vi "Write Direction.vi"(10 "Velocity":T1, 11 "Flying Saucer in":refnum<class "Flying Saucer.lvclass">) -> (3 "Flying Saucer out":refnum<class "Flying Saucer.lvclass">)   [LabVIEW 2024, in "Flying Saucer.lvclass"]
doc: "MIT Licence\nCopyright (c) 2024 David Grollier"
uses:
  Flying Saucer.lvclass
  Type Def/Velocity.ctl
  Flying Saucer.lvclass/Flying Saucer.ctl
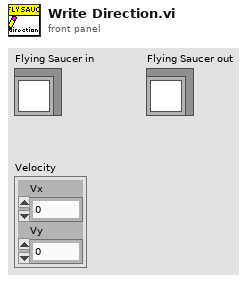
[diagram p1: front panel]
types:
  T1 = typedef "Velocity.ctl" = cluster{"Vx":dbl, "Vy":dbl}
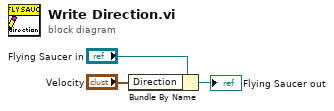
[diagram p0: block diagram]
diagram:
  n1 = Bundle By Name(cluster="Flying Saucer in", "Direction"="Velocity") -> (→"Flying Saucer out":refnum<class "Flying Saucer.lvclass">)
